vi "line flow cluster to 1d array.vi"(1 "Flowrate Data":T1(array[cluster])) -> (0 "Array":dbl[](array[numeric]))   [LabVIEW 2018]
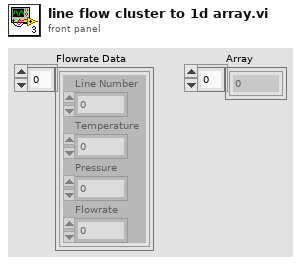
[diagram p1: front panel]
types:
  T1 = cluster{"Line Number":dbl, "Temperature":dbl, "Pressure":dbl, "Flowrate":dbl}[]
  T2 = cluster{"Line Number":dbl, "Temperature":dbl, "Pressure":dbl, "Flowrate":dbl}
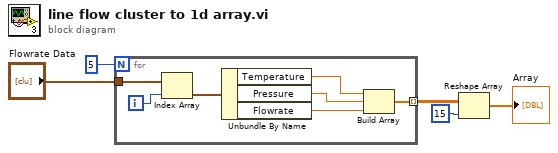
[diagram p0: block diagram]
diagram:
  n1 = for {
    N: 5 -> [_]
    tunnel: "Flowrate Data" -> [w12]
    tunnel: [w6] -> w3 mode=indexing
    i -> [w11]
    n2 = Index Array(array=w12, index=w11) -> (element=w10:T2)
    n3 = Unbundle By Name(w10) -> ("Temperature"=w9:dbl, "Pressure"=w8:dbl, "Flowrate"=w7:dbl)
    n4 = Build Array(w9, w8, w7) -> (w6:dbl[])
  }
  n5 = Reshape Array(w3, 15 ("dimension size")) -> (→"Array":dbl[])
